vi "Write Port.vi"(0 "Serial Device in":refnum<class "Serial Device.lvclass">, 5 "VISA resource name":refnum<visa-resource-name>, 9 "Port":u16, 11 "error in (no error)":errorcluster, 12 "Set Port":bool[](array[boolean])) -> (4 "Serial Device out":refnum<class "Serial Device.lvclass">, 6 "VISA resource name out":refnum<visa-resource-name>, 15 "error out":errorcluster)   [LabVIEW 2020, in "Serial Device.lvclass"]
uses:
  Serial Device.lvclass
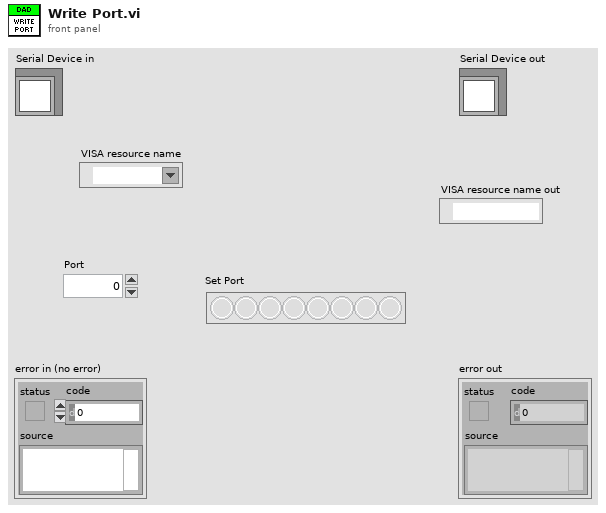
[diagram p1: front panel]
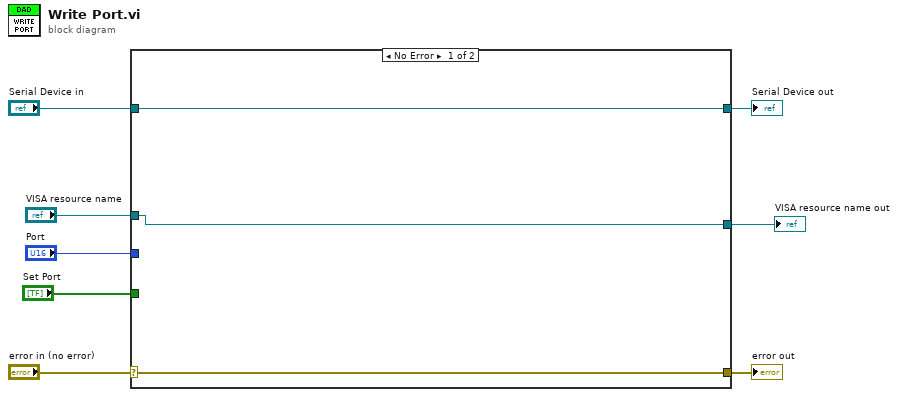
[diagram p0: block diagram]
diagram:
  n1 = case shown="No Error" "error in (no error)" {
    selector: "error in (no error)" -> [w10 w14]
    tunnel: [w10 w14] -> w7
    tunnel: [w11 w13] -> w5
    tunnel: "Serial Device in" -> [w11 w13]
    tunnel: "VISA resource name" -> [w9 w12]
    tunnel: [w9 w12] -> w3
    tunnel: "Port" -> [_ _]
    tunnel: "Set Port" -> [_ _]
    frame No Error {
    }
    frame Error {
    }
  }
  "error out" <- w7
  "Serial Device out" <- w5
  "VISA resource name out" <- w3
